vi "ZCAN_Filter.vi"(7 "error in (no error)":errorcluster caption="错误输入（无错误）", 8 "Filter":T1 {"Config"."End" format="%x"; "Config"."Start" format="%x"}, 10 "channel_handle":u32) -> (0 "error out":errorcluster caption="错误输出")   [LabVIEW 2011, in "zlgcan.lvlib"]
doc: "设置滤波，最多设置50条\n在SubVI内部设置，可根据项目实际需求修改\n在Init 初始化之后， Start 之前使用\n\n适用型号：USBCANFD-100U、USBCANFD-200U、USBCANFD-MINI、\nPCI-5010-U、PCI-5020-U、USBCAN-E-U、USBCAN-2E-U、CANalyst-II+、\nUSBCAN-4E-U"
uses:
  zlgcan.lvlib
panel:
  # "在后面板添加滤波表格"
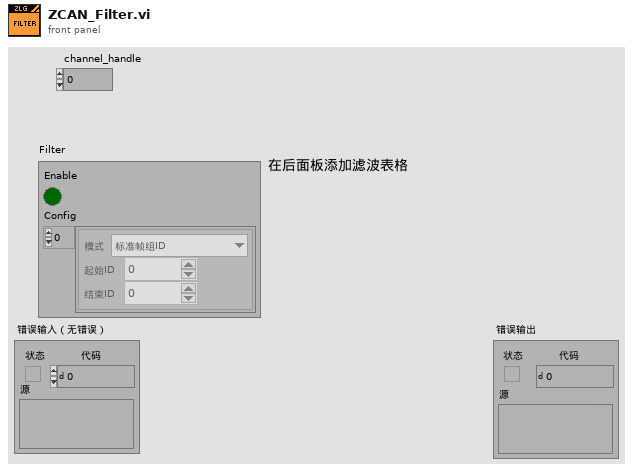
[diagram p1: front panel]
types:
  T1 = cluster{"Enable":bool, "Config":cluster{"Mode":enum16{"标准帧组ID", "标准帧明确ID", "扩展帧组ID", "扩展帧明确ID"}, "Start":u32, "End":u32}[]}
  T2 = cluster{"Mode":enum16{"标准帧组ID", "标准帧明确ID", "扩展帧组ID", "扩展帧明确ID"}, "Start":u32, "End":u32}[]
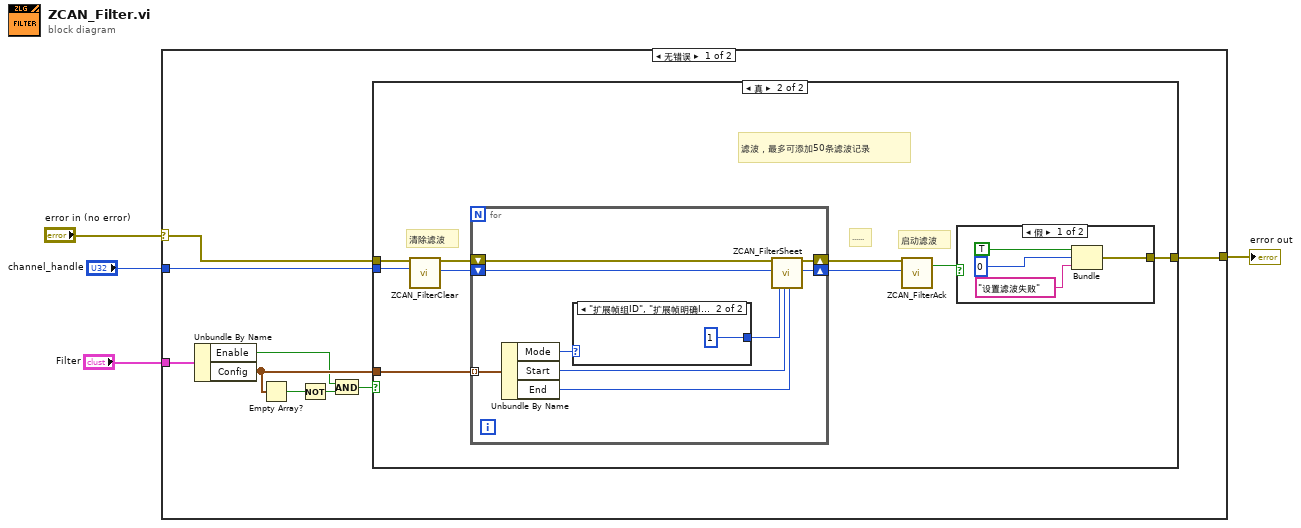
[diagram p0: block diagram]
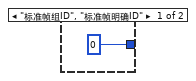
[diagram p3: hidden frame]
diagram:
  n1 = case shown="无错误" "error in (no error)" {
    selector: "error in (no error)" -> [w12 w39]
    tunnel: [w13 w39] -> w3
    tunnel: "channel_handle" -> [w11 _]
    tunnel: "Filter" -> [w10 _]
    frame No Error {
      n2 = Unbundle By Name(w10) -> ("Enable"=w6:bool, "Config"=w9:T2)
      n3 = Empty Array?(array=w9) -> (empty?=w8:bool)
      n4 = Not(x=w8) -> (.not. x?=w7:bool)
      n5 = And(x=w6, y=w7) -> (x .and. y?=w5:bool)
      n6 = case shown="真" w5 {
        tunnel: [w14 w23] -> w13
        tunnel: w12 -> [w14 w22]
        tunnel: w11 -> [_ w21]
        tunnel: w9 -> [_ w15]
        frame False {
        }
        frame True {
          # "......"
          # "启动滤波"
          # "清除滤波"
          # "滤波，最多可添加50条滤波记录"
          n7 = call "ZCAN_FilterClear.vi"("error in (no error)"=w22, "can_index_handle"=w21) -> ("error out"=w19:errorcluster, "can_index_handle(out)"=w17:u32)  [unwired: 16 in]
          n8 = for {
            shift-right: [w31] -> w18
            shift-left: w19 -> [w32]
            shift-right: [w29] -> w16
            shift-left: w17 -> [w30]
            tunnel: w15 -> [w28] mode=indexing
            n9 = Unbundle By Name(w28) -> ("Mode"=w27:enum16{"标准帧组ID", "标准帧明确ID", "扩展帧组ID", "扩展帧明确ID"}, "Start"=w25:u32, "End"=w24:u32)
            n10 = case shown="\"扩展帧组ID\", \"扩展帧明确ID\"" w27 {
              tunnel: [u32 0 ("filter_mode") u32 1 ("filter_mode")] -> w26
              frame "标准帧组ID", "标准帧明确ID" {
              }
              frame "扩展帧组ID", "扩展帧明确ID" {
              }
            }
            n11 = call "ZCAN_FilterSheet.vi"("error in (no error)"=w32, "can_index_handle"=w30, "filter_mode"=w26, "Start"=w25, "End"=w24) -> ("error out"=w31:errorcluster, "can_index_handle（out）"=w29:u32)  [unwired: 13 in]
          }
          n12 = call "ZCAN_FilterAck.vi"("error in (no error)"=w18, "can_index_handle"=w16) -> ("启动滤波成功？"=w20:bool)  [unwired: 15 in, 2 out]
          n13 = case shown="假" w20 {
            tunnel: [w35 _] -> w23
            frame False {
              n14 = Bundle("status"=TRUE, "code"=0, "消息"="设置滤波失败") -> (w35:cluster{"status":bool, "code":i32, "消息":string})  [unwired: 1 in]
            }
            frame True {
            }
          }
        }
      }
    }
    frame Error {
    }
  }
  "error out" <- w3
